vi "Dashboard Main.vi"() -> ()   [LabVIEW 2018]
uses:
  <vilib>/Rock Robotics/Network Tables/NT Read Numeric Array.vi
  <vilib>/Rock Robotics/Network Tables/NT Write Boolean.vi
  <vilib>/Rock Robotics/Network Tables/NT Write Number.vi
panel:
  out "Camera Perf":string
  in  "Camera Settings":T1={"Frame Rate"=30, "Compression"=30, "Size"=1, "DB Camera Config"=FALSE} {"Frame Rate" scale=1.0..30.0; "Compression" scale=100.0..-1.0; "Size" items=["640x480", "320x240", "160x120"]}
  in  "TCP":refnum<k5>
  out "Robot IP":string
  in  "Dashboard Tab":enum32{"Drive", "Basic", "Custom", "Variables"}(tab)
  in  "Select Auto":string(combo)="Select Autonomous ..."
  out "NT Connection":bool
  out "MotorChart R":cluster{"Numeric":dbl, "Numeric":dbl}(graph)
  out "MotorChart L":cluster{"Numeric":dbl, "Numeric":dbl}(graph)
  out "MotorSliders R":cluster{"MotorSlide1":dbl, "MotorSlide2":dbl} {"MotorSlide2" scale=-1.0..1.0 scale format="%#_2e"; "MotorSlide1" scale=-1.0..1.0 scale format="%#_2e"}
  out "MotorSliders L":cluster{"MotorSlide1":dbl, "MotorSlide2":dbl} {"MotorSlide2" scale=-1.0..1.0 scale format="%#_2e"; "MotorSlide1" scale=-1.0..1.0 scale format="%#_2e"}
  out "JS1 Z":dbl(slide) scale=-1.0..1.0 scale format="%#_2e"
  out "JS1 Graph":cluster{"X":dbl, "Y":dbl}[](graph)
  out "JS1 Buttons":T2
  out "JS2 Z":dbl(slide) scale=-1.0..1.0 scale format="%#_2e"
  out "JS2 Graph":cluster{"X":dbl, "Y":dbl}[](graph)
  out "JS2 Buttons":T2
  out "Mode":T3(ring)=enum."Auto Disabled"
  in  "Driving Enabled":bool
  in  "Arcade Drive":bool
  in  "Speed":dbl
  in  "DB/String 9":string
  in  "DB/String 8":string
  in  "DB/String 7":string
  in  "DB/String 6":string
  in  "DB/String 5":string
  in  "DB/String 4":string
  in  "DB/String 3":string
  in  "DB/String 2":string
  in  "DB/String 1":string
  in  "DB/String 0":string
  in  "DB/Slider 0":dbl(slide) scale=0.0..5.0
  in  "DB/Slider 1":dbl(slide) scale=0.0..5.0
  in  "DB/Slider 2":dbl(slide) scale=0.0..5.0
  in  "DB/Slider 3":dbl(slide) scale=0.0..5.0
  out "DB/LED 3":bool
  out "DB/LED 2":bool
  out "DB/LED 1":bool
  out "DB/LED 0":bool
  in  "DB/Button 3":bool
  in  "DB/Button 2":bool
  in  "DB/Button 1":bool
  in  "DB/Button 0":bool caption="New Name"
  out "Tree":string(tree)
  out "Camera Image":T4(plugin-control)
  out "Background":bool
  in  "Camera Name":string(combo)="No Camera Selection"
  # "HW"
  # "Joysticks"
  # "Drive Motors"
  # "Front"
  # "Right"
  # "Left"
  # "Back"
  # "This tab is a great place for autonomous settings and robot-specific values.\nPlace controls and indicators inside this tab and match name to\nDashboard Variables on robot. You can also delete this comment."
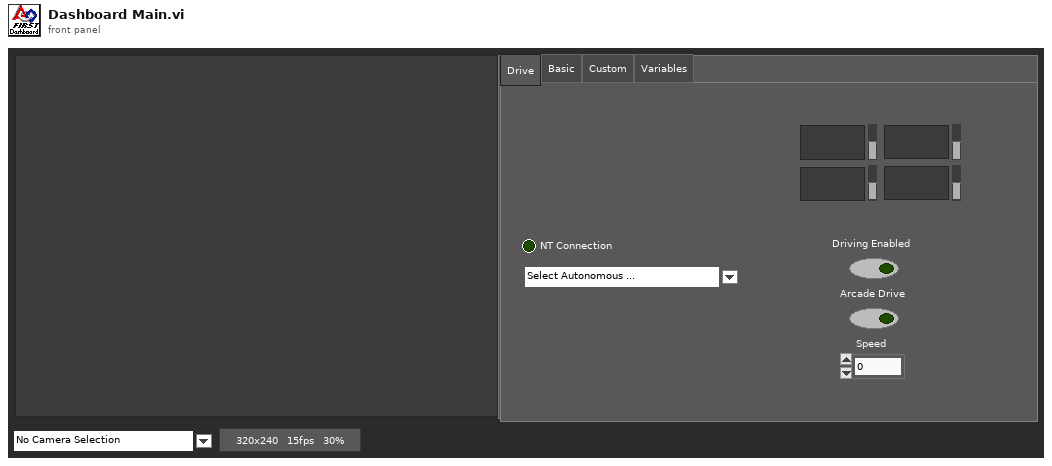
[diagram p1: front panel]
types:
  T1 = cluster{"Frame Rate":i32, "Compression":i32, "Size":u16, "DB Camera Config":bool}
  T2 = cluster{bool, bool, bool, bool, bool, bool, bool, bool, bool, bool, bool, bool}
  T3 = enum8{"Tele-Op Disabled", "Tele-Op Enabled", "Auto Disabled", "Auto Enabled", "Test Disabled", "Test Enabled", "Disconnected", "No Code", "E-Stop"}
  T4 = typedef "IMAQ Image.ctl" = refnum<image>
  T5 = cluster{"Save Path":path, "Interval (s)":dbl, "Keep":i32}
  T6 = typedef "Image Type" = u32
  T7 = cluster{"Camera Image":refnum<vi>, "Dashboard Tab":refnum<vi>, "Background":refnum<vi>, "Tree":refnum<vi>, "Camera Settings":refnum<vi>, "Camera Name":refnum<vi>, "Camera Perf":refnum<vi>}
  T8 = cluster{"Error Strings":string, "Disable Counts":cluster{u16, u16}, "Rail Faults":cluster{u16, u16, u16}, "Robot IP":string, "DB Mode":u8, "Event Info":cluster{"Name":string, "Type":u8, "Number":u16, "Replay":u8}}
  T9 = cluster{"Storage":cluster{"Disk Free":u64, "RAM Block":u32, "RAM free":u32}, "CPU Utilization":cluster{"CPU % ISR":sgl, "CPU % Time Crit":sgl, "CPU % Timed Str":sgl, "CPU % High":sgl, "CPU % Above":sgl, "CPU % Normal":sgl, "CPU % Low":sgl}, "CAN":cluster{"% Bus Utilization":sgl, "Bus Off Cnt":u32, "TX_FIFO Full Cnt":u32, "Receive Error Cnt":u8, "Transmit Error Cnt":u8}, "HID":cluster{"HID Outputs":u32, "Rumble Low":u16, "Rumble High":u16}[]}
  T10 = cluster{"Status bits":cluster{"Test Mode":bool, "Autonomous":bool, "Enabled":bool, "Code Start":bool, "Brownout":bool, "Reserved 2":bool, "Reserved 3":bool, "E-Stop":bool}, "Code Trace":cluster{"Disabled":bool, "TeleOp":bool, "Auto":bool, "Test":bool}, "Controller Type":enum16{"unknown", "cRIO", "roboRio"}, "Code?":enum16{"unknown", "noCode", "code"}, "Battery V":dbl}
  T11 = cluster{"Control Bits":cluster{"TestMode":bool, "Autonomous":bool, "Enabled":bool, "FMS Present":bool, bool, bool, bool, "E-Stop":bool}, "Team Station ":u8, "Countdown":sgl, "Joystick Values":cluster{"Axes":dbl[], "Buttons":bool[], "POVs":i16[]}[]}
  T12 = cluster{"Axes":dbl[], "Buttons":bool[], "POVs":i16[]}[]
  T13 = cluster{"Axes":dbl[], "Buttons":bool[], "POVs":i16[]}
  T14 = cluster{"Buttons[0]":bool, "Buttons[1]":bool, "Buttons[2]":bool, "Buttons[3]":bool, "Buttons[4]":bool, "Buttons[5]":bool, "Buttons[6]":bool, "Buttons[7]":bool, "Buttons[8]":bool, "Buttons[9]":bool, "Buttons[10]":bool, "Buttons[11]":bool}
  T15 = cluster{"Shift":bool, "Ctrl":bool, "Alt":bool, "Cmd":bool, "Opt":bool}
  T16 = cluster{"Camera Name":string, "Camera File Name":string, "Saved DB Images Info":cluster{"Save Path":path, "Interval (s)":dbl, "Keep":i32}}
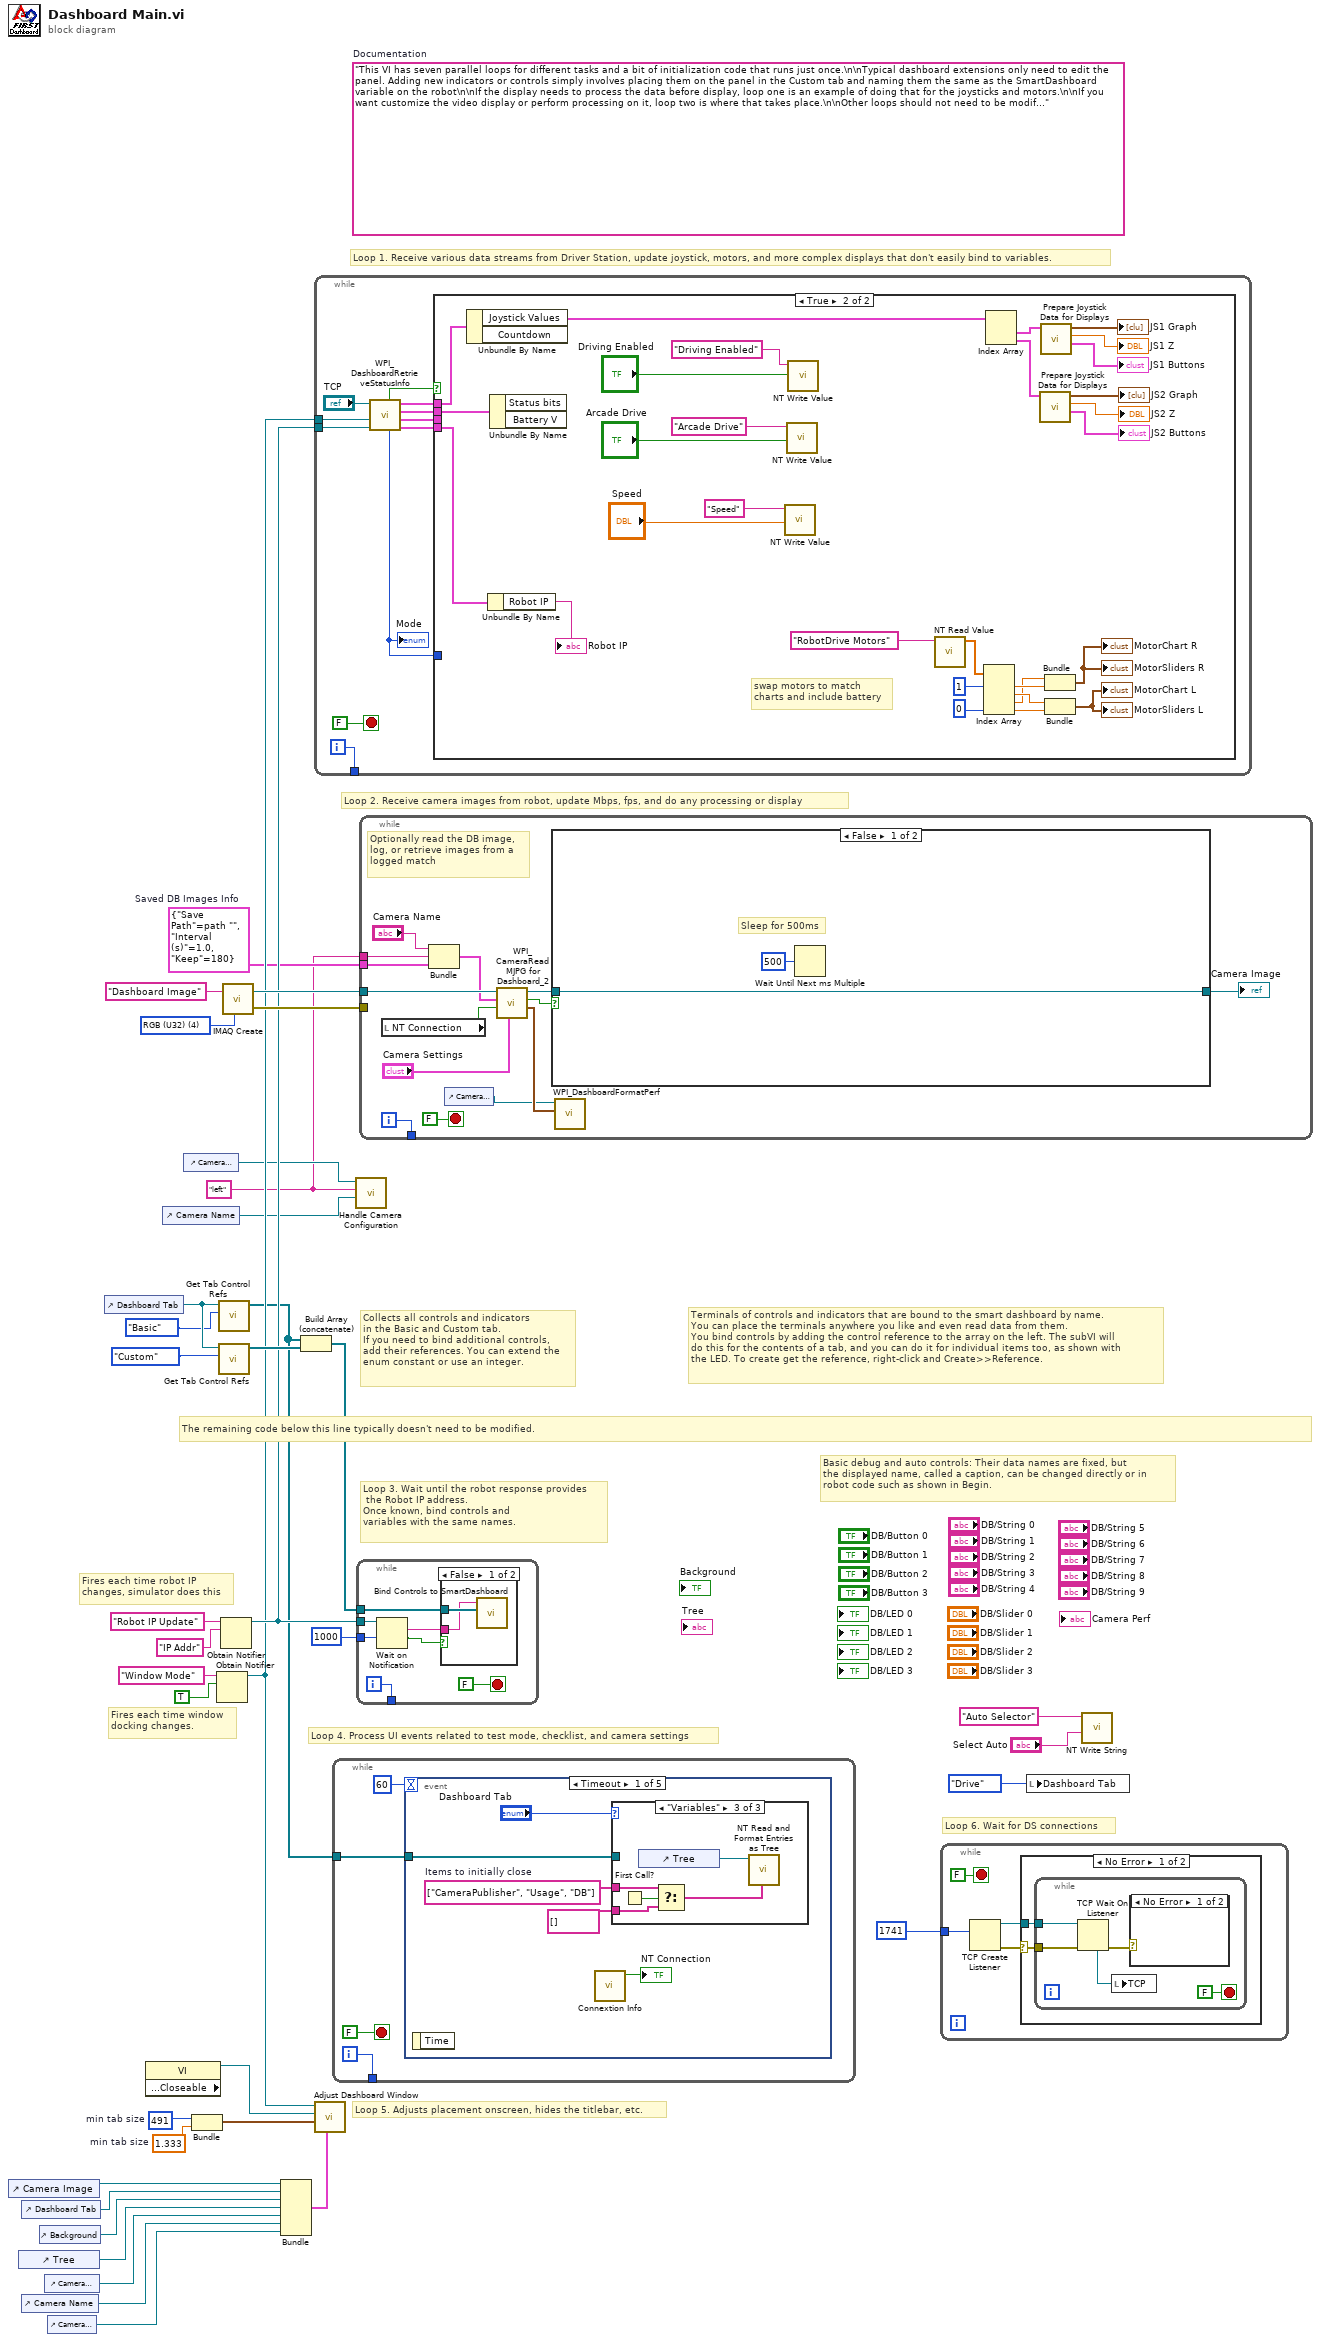
[diagram p0: block diagram]
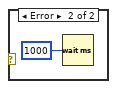
[diagram p2: hidden frame]
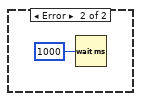
[diagram p3: hidden frame]
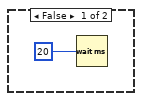
[diagram p4: hidden frame]
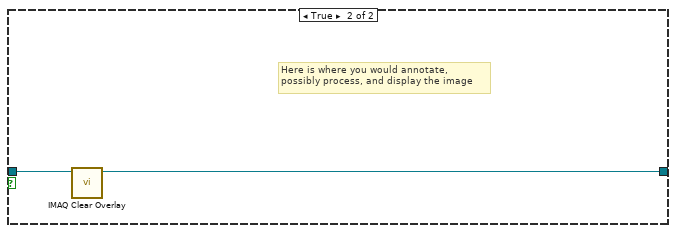
[diagram p6: hidden frame]
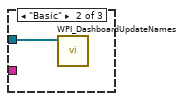
[diagram p8: hidden frame]
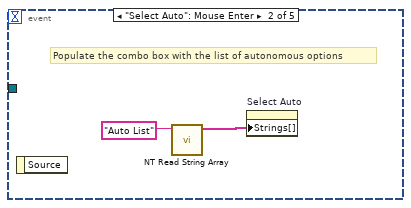
[diagram p9: hidden frame]
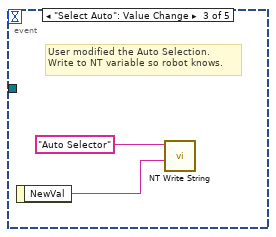
[diagram p10: hidden frame]
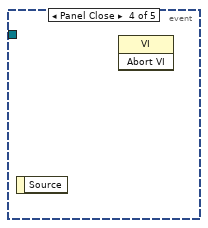
[diagram p11: hidden frame]
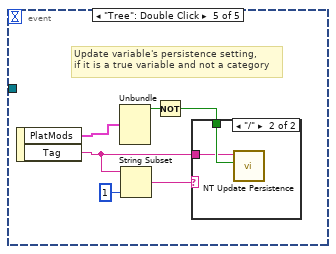
[diagram p12: hidden frame]
diagram:
  w1 = "left" ("Camera File Name")
  w2 = T5 {"Save Path"=path "", "Interval (s)"=1.0, "Keep"=180}  # Saved DB Images Info
  w22 = 491  # min tab size
  w21 = 1.333  # min tab size
  (unwired) "This VI has seven parallel loops for different tasks and a bit of initialization code that runs just once.\n\nTypical dashboard extensions only need to edit the panel. Adding new indicators or controls simply involves placing them on the panel in the Custom tab and naming them the same as the SmartDashboard variable on the robot\n\nIf the display needs to process the data before display, loop one is an example of doing that for the joysticks and motors.\n\nIf you want customize the video display or perform processing on it, loop two is where that takes place.\n\nOther loops should not need to be modified. They are pretty standard, and document the task they perform."  # Documentation
  w37 = T6 4 items=["Grayscale (U8)", "Grayscale (I16)", "Grayscale (SGL)", "Complex (CSG)", "RGB (U32)", "HSL (U32)", "RGB (U64)"] ("Image Type")
  # "Loop 6. Wait for DS connections"
  # "Basic debug and auto controls: Their data names are fixed, but\nthe displayed name, called a caption, can be changed directly or in\nrobot code such as shown in Begin."
  # "Fires each time robot IP\nchanges, simulator does this"
  # "Fires each time window\ndocking changes."
  # "Collects all controls and indicators\nin the Basic and Custom tab.\nIf you need to bind additional controls,\nadd their references. You can extend the\nenum constant or use an integer."
  # "The remaining code below this line typically doesn't need to be modified."
  # "Loop 4. Process UI events related to test mode, checklist, and camera settings"
  # "Terminals of controls and indicators that are bound to the smart dashboard by name.\nYou can place the terminals anywhere you like and even read data from them.\nYou bind controls by adding the control reference to the array on the left. The subVI will\ndo this for the contents of a tab, and you can do it for individual items too, as shown with\nthe LED. To create get the reference, right-click and Create>>Reference."
  # "Loop 3. Wait until the robot response provides\n the Robot IP address.\nOnce known, bind controls and\nvariables with the same names."
  # "Loop 5. Adjusts placement onscreen, hides the titlebar, etc."
  # "Loop 1. Receive various data streams from Driver Station, update joystick, motors, and more complex displays that don't easily bind to variables."
  # "Loop 2. Receive camera images from robot, update Mbps, fps, and do any processing or display"
  n1 = control-ref of="Camera Image"() -> (w24:refnum<vi>)
  n2 = control-ref of="Tree"() -> (w8:refnum<vi>)
  n3 = control-ref of="Dashboard Tab"() -> (w23:refnum<vi>)
  n4 = control-ref of="Camera Name"() -> (w6:refnum<vi>)
  n5 = control-ref of="Background"() -> (w19:refnum<vi>)
  n6 = control-ref of="Camera Settings"() -> (w7:refnum<vi>)
  n7 = control-ref of="Camera Perf"() -> (w5:refnum<vi>)
  n8 = control-ref of="Dashboard Tab"() -> (w27:refnum<vi>)
  n9 = property class="VI" props=["Front Panel.Closeable"]() -> (reference out=w28:refnum<vi>)  [unwired: 2 in, 2 out]
  n10 = control-ref of="Camera Name"() -> (w12:refnum<vi>)
  n11 = control-ref of="Camera Settings"() -> (w13:refnum<vi>)
  n12 = Bundle("min tab size"=w22, "min tab size"=w21) -> (w20:cluster{"min tab size":i32, "min tab size":dbl})  [unwired: 1 in]
  n13 = Obtain Notifier(name (unnamed)="Window Mode", notification data type=TRUE) -> (notifier out=w16:refnum<notifier>)  [unwired: 2 in, 2 out]
  n14 = call <vilib>:"Get Tab Control Refs.vi"("Page Index"=enum32{"Drive", "Basic", "Custom", "Variables"}."Basic" ("Dashboard Tab"), "TabControl in"=w27) -> ("ControlsOnPage"=w11:refnum<vi>[])  [unwired: 9 in]
  n15 = call <vilib>:"Get Tab Control Refs.vi"("Page Index"=enum32{"Drive", "Basic", "Custom", "Variables"}."Custom" ("Dashboard Tab"), "TabControl in"=w27) -> ("ControlsOnPage"=w26:refnum<vi>[])  [unwired: 9 in]
  n16 = Obtain Notifier(name (unnamed)="Robot IP Update", notification data type="IP Addr" ("name (unnamed)")) -> (notifier out=w17:refnum<notifier>)  [unwired: 2 in, 2 out]
  n17 = call "IMAQ Create"("Image Name"="Dashboard Image", "Image Type"=w37) -> ("New Image"=w35:T4, "error out"=w34:errorcluster)  [unwired: 2 in, 1 out]
  n18 = Bundle("Camera Image"=w24, "Dashboard Tab"=w23, "Background"=w19, "Tree"=w8, "Camera Settings"=w7, "Camera Name"=w6, "Camera Perf"=w5) -> (w18:T7)  [unwired: 1 in]
  n19 = Build Array (concatenate)(w11, w26) -> (w25:refnum<vi>[])
  n20 = while {
    tunnel: [w47] -> _
    tunnel: w17 -> [w41]
    tunnel: w16 -> [w38]
    i -> [w47]
    stop <- FALSE stop-if-true
    n21 = call <vilib>:"WPI_DashboardRetrieveStatusInfo.vi"("Binding Refnum"=w41, "Window Mode Notifier"=w38, "TCP Cnx"="TCP") -> ("Power and Errors"=w42:T8, "Robot Metrics"=w45:T9, "Status Info"=w46:T10, "Control Info"=w43:T11, "Robot Mode"=w40:T3, "Process?"=w44:bool)  [unwired: 3 in]
    "Mode" <- w40
    n22 = case shown="True" w44 {
      tunnel: w46 -> [_ w78]
      tunnel: w45 -> [_ _]
      tunnel: w43 -> [_ w77]
      tunnel: w42 -> [_ w76]
      tunnel: w40 -> [_ _]
      frame False {
        n23 = Wait (ms)(milliseconds to wait=u32 20) -> ()  [unwired: 1 out]
      }
      frame True {
        # "swap motors to match\ncharts and include battery"
        n24 = Unbundle By Name(w77) -> ("Joystick Values"=w67:T12)  [unwired: 1 out]
        n25 = Unbundle By Name(w76) -> ("Robot IP"=→"Robot IP":string)
        n26 = Unbundle By Name(w78) -> ()  [unwired: 2 out]
        n27 = call-poly <vilib>:"NT Write Value.vi"("Numeric"="Speed", "Name"="Speed") -> ()  [unwired: 9 in, 1 out]
        n28 = call-poly <vilib>:"NT Write Value.vi"("Boolean"="Arcade Drive", "Name"="Arcade Drive") -> ()  [unwired: 9 in, 1 out]
        n29 = call-poly <vilib>:"NT Write Value.vi"("Boolean"="Driving Enabled", "Name"="Driving Enabled") -> ()  [unwired: 9 in, 1 out]
        n30 = call-poly <vilib>:"NT Read Value.vi"("Name"="RobotDrive Motors") -> ("Numeric Array"=w57:dbl[])  [unwired: 9 in, 1 out]
        n31 = Index Array(array=w57, index #1=1, index #4=0) -> (element #1=w71:dbl, element #2=w72:dbl, element #3=w70:dbl, element #4=w75:dbl)  [unwired: 2 in]
        n32 = Index Array(array=w67) -> (element #1=w66:T13, element #2=w62:T13)  [unwired: 2 in]
        n33 = call "Prepare Joystick Data for Displays.vi"("Joystick Values"=w62) -> ("Buttons"=→"JS2 Buttons":T14, "Z Axis"=→"JS2 Z":dbl, "Cartesian Data"=→"JS2 Graph":cluster{"X axis":dbl, "X axis":dbl}[])  [unwired: 8 in]
        n34 = call "Prepare Joystick Data for Displays.vi"("Joystick Values"=w66) -> ("Buttons"=→"JS1 Buttons":T14, "Z Axis"=→"JS1 Z":dbl, "Cartesian Data"=→"JS1 Graph":cluster{"X axis":dbl, "X axis":dbl}[])  [unwired: 8 in]
        n35 = Bundle("Numeric"=w70, "Numeric"=w71) -> (→"MotorChart R" →"MotorSliders R":cluster{"Numeric":dbl, "Numeric":dbl})  [unwired: 1 in]
        n36 = Bundle("Numeric"=w72, "Numeric"=w75) -> (→"MotorChart L" →"MotorSliders L":cluster{"Numeric":dbl, "Numeric":dbl})  [unwired: 1 in]
      }
    }
  }
  n37 = call "Adjust Dashboard Window.vi"("Sizing Refnums"=w18, "Size Constraints"=w20, "VI"=w28, "WIn Mode"=w16) -> ()  [unwired: 8 in]
  n38 = while {
    tunnel: [w80] -> _
    tunnel: w11 -> [w79]
    i -> [w80]
    stop <- FALSE stop-if-true
    n39 = event shown="[0] Timeout" {
      selector: _ -> [_ _ _ _ _]
      dyn-events: _ -> [_ _ _ _ _]
      timeout: u32 60 ("milliseconds to wait") -> [_ _ _ _ _]
      tunnel: w79 -> [w85 _ _ _ _]
      event Timeout {
        w84 = string[] ["CameraPublisher", "Usage", "DB"]  # Items to initially close
        n40 = event-data() -> ()  [unwired: 1 in, 1 out]
        n41 = call <vilib>:"Connextion Info.vi"() -> ("Connected"=→"NT Connection":bool)  [unwired: 10 in, 1 out]
        n42 = case shown="\"Variables\"" "Dashboard Tab" {
          tunnel: w85 -> [_ w88 _]
          tunnel: w84 -> [_ _ w91]
          tunnel: string[] [] -> [_ _ w90]
          frame "Custom", Default {
          }
          frame "Basic" {
            n43 = call <vilib>:"WPI_DashboardUpdateNames.vi"("Controls on Tab"=w88) -> ()  [unwired: 11 in]
          }
          frame "Variables" {
            n44 = First Call?() -> (First Call?: T/F=w92:bool)
            n45 = control-ref of="Tree"() -> (w93:refnum<vi>)
            n46 = Select(t=w91, s=w92, f=w90) -> (s? t:f=w89:string[])
            n47 = call <vilib>:"NT Read and Format Entries as Tree.vi"("Tags to  Close"=w89, "Tree Refnum"=w93) -> ()  [unwired: 8 in, 2 out]
          }
        }
      }
      event "Select Auto": Mouse Enter {
        # "Populate the combo box with the list of autonomous options"
        n48 = event-data() -> ()  [unwired: 1 in, 1 out]
        n49 = call <vilib>:"NT Read String Array.vi"("Name"="Auto List") -> ("String Array"=w94:string[])  [unwired: 9 in, 1 out]
        n50 = property on="Select Auto" class="CmbBox"("Strings[]"=w94) -> ()  [unwired: 2 in, 2 out]
      }
      event "Select Auto": Value Change {
        # "User modified the Auto Selection.\nWrite to NT variable so robot knows."
        n51 = event-data() -> ("NewVal"=w96:string)  [unwired: 1 in]
        n52 = call <vilib>:"NT Write String.vi"("String"=w96, "Name"="Auto Selector") -> ()  [unwired: 9 in, 1 out]
      }
      event Panel Close {
        n53 = event-data() -> ()  [unwired: 1 in, 1 out]
        n54 = invoke class="VI" method="Abort VI"() -> ()  [unwired: 3 in, 3 out]
      }
      event "Tree": Double Click {
        # "Update variable's persistence setting,\nif it is a true variable and not a category"
        n55 = event-data() -> ("PlatMods"=w99:T15, "Tag"=w98:string)  [unwired: 1 in]
        n56 = Unbundle(w99) -> ("Shift"=w103:bool)  [unwired: 4 out]
        n57 = String Subset(string=w98, length (rest)=1 ("length (rest)")) -> (substring=w100:string)  [unwired: 1 in]
        n58 = Not(x=w103) -> (.not. x?=w102:bool)
        n59 = case shown="\"/\"" w100 {
          tunnel: w102 -> [_ w105]
          tunnel: w98 -> [_ w104]
          frame Default {
          }
          frame "/" {
            n60 = call <vilib>:"NT Update Persistence.vi"("Persistence"=w105, "Name"=w104) -> ()  [unwired: 9 in, 1 out]
          }
        }
      }
    }
  }
  n61 = call "Handle Camera Configuration.vi"("CameraNameRef"=w12, "Display Name"=w1, "ClusterRef"=w13) -> ()  [unwired: 9 in]
  n62 = while {
    tunnel: w25 -> [w112]
    tunnel: w17 -> [w110]
    tunnel: [w108] -> _
    tunnel: u32 1000 ("milliseconds to wait") -> [w107]
    i -> [w108]
    stop <- FALSE stop-if-true
    n63 = Wait on Notification(notifier=w110, timeout in ms (-1)=w107) -> (notification=w109:string, timed out?=w106:bool)  [unwired: 2 in, 2 out]
    n64 = case shown="False" w106 {
      tunnel: w112 -> [w114 _]
      tunnel: w109 -> [w113 _]
      frame False {
        n65 = call <vilib>:"Bind Controls to SmartDashboard.vi"("Bound Control Refs"=w114, "Server IP Address"=w113) -> ()  [unwired: 10 in]
      }
      frame True {
      }
    }
  }
  n66 = while {
    tunnel: w35 -> [w126]
    tunnel: w34 -> [_]
    tunnel: [w127] -> _
    tunnel: w2 -> [w120]
    tunnel: w1 -> [w117]
    i -> [w127]
    stop <- FALSE stop-if-true
    # "Optionally read the DB image,\nlog, or retrieve images from a\nlogged match"
    n67 = local read "NT Connection"() -> (w121:bool)
    n68 = Bundle("Camera Name"="Camera Name", "Camera File Name"=w117, "Saved DB Images Info"=w120) -> (w119:T16)  [unwired: 1 in]
    n69 = control-ref of="Camera Perf"() -> (w115:refnum<vi>)
    n70 = call <vilib>:"WPI_CameraRead MJPG for Dashboard_2.vi"("Camera Settings"="Camera Settings", "NT Connection"=w121, "Capture Info"=w119, "Image in"=w126) -> ("perf info"=w116:cluster{"Bandwidth (Mbps)":dbl, "fps":dbl}, "Active"=w124:bool, "Image\\ out"=w125:T4)  [unwired: 5 in]
    n71 = case shown="False" w124 {
      tunnel: w125 -> [w129 w132]
      tunnel: [w129 w131] -> w122
      frame False {
        # "Sleep for 500ms"
        n72 = Wait Until Next ms Multiple(millisecond multiple=u32 500) -> ()  [unwired: 1 out]
      }
      frame True {
        # "Here is where you would annotate,\npossibly process, and display the image"
        n73 = call "IMAQ Clear Overlay"("Image"=w132) -> ("Image Out"=w131:T4)  [unwired: 2 in, 8 out]
      }
    }
    "Camera Image" <- w122
    n74 = call <vilib>:"WPI_DashboardFormatPerf.vi"("Performance"=w116, "String in"=w115) -> ()  [unwired: 10 in]
  }
  n75 = while {
    tunnel: u16 1741 ("timeout ms (25000)") -> [w134]
    stop <- FALSE stop-if-true
    n76 = TCP Create Listener(10:w134) -> (0:w133:errorcluster, 3:w135:refnum<k5>)  [unwired: 4 in, 1 out]
    n77 = case shown="No Error" w133 {
      selector: w133 -> [w137 _]
      tunnel: w135 -> [w138 _]
      frame No Error {
        n78 = while {
          tunnel: w138 -> [w141]
          tunnel: w137 -> [w140]
          stop <- FALSE stop-if-true
          n79 = TCP Wait On Listener(8:w140, 11:w141) -> (0:w142:errorcluster, 4:w143:refnum<k5>)  [unwired: 2 in, 3 out]
          n80 = local write "TCP"(w143) -> ()
          n81 = case shown="No Error" w142 {
            frame No Error {
            }
            frame Error {
              n82 = Wait (ms)(milliseconds to wait=u32 1000) -> ()  [unwired: 1 out]
            }
          }
        }
      }
      frame Error {
        n83 = Wait (ms)(milliseconds to wait=u32 1000) -> ()  [unwired: 1 out]
      }
    }
  }
  n84 = local write "Dashboard Tab"(enum32{"Drive", "Basic", "Custom", "Variables"}."Drive" ("Dashboard Tab")) -> ()
  n85 = call <vilib>:"NT Write String.vi"("String"="Select Auto", "Name"="Auto Selector") -> ()  [unwired: 9 in, 1 out]
